vi "FL_Decode_RAW_to_DEC_for_saving.vi"(0 "Sensor board size":string="Small", 1 "IO ports config":bool[](array[boolean])=[TRUE, TRUE, FALSE, FALSE], 2 "Input timestamp":timestamp, 3 "Input string":string, 4 "IO inversion config.":u16, 5 "Error In":errorcluster) -> (6 "Output string leftover":string, 7 "DEC output cluster":T1, 8 "Error Out":errorcluster)   [LabVIEW 2018, in "Tracker.lvlib"]
uses:
  Tracker.lvlib
panel:
  out "TTL ins":bool[](array[boolean])
  out "TTL outs":bool[](array[boolean])
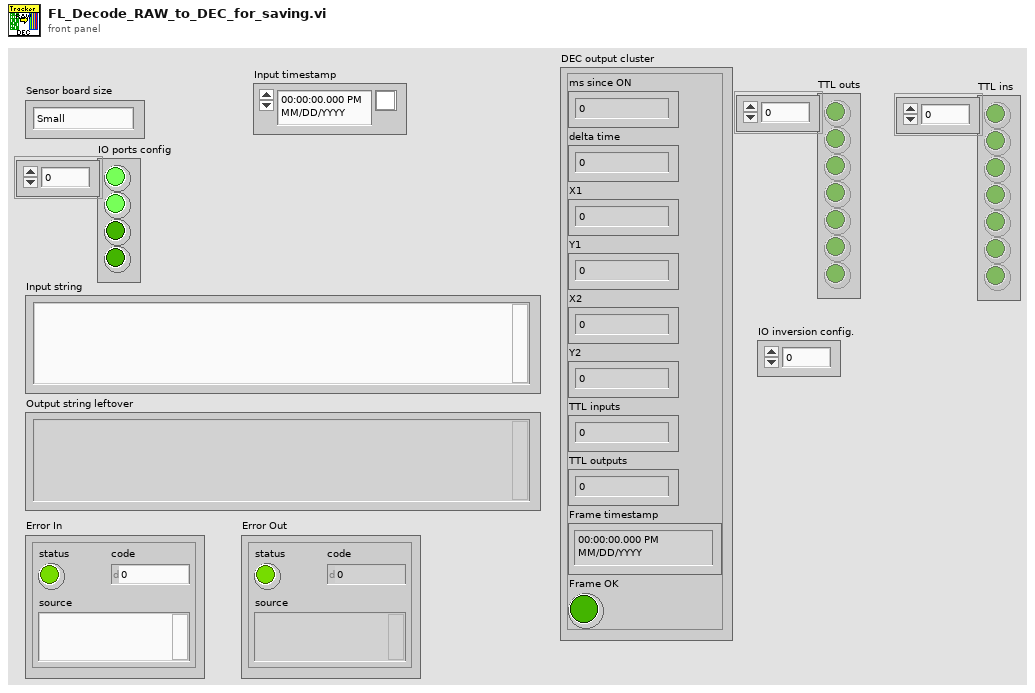
[diagram p1: front panel]
types:
  T1 = cluster{"ms since ON":u32, "delta time":u32, "X1":sgl, "Y1":sgl, "X2":sgl, "Y2":sgl, "TTL inputs":u8, "TTL outputs":u8, "Frame timestamp":timestamp, "Frame OK":bool}
  T2 = cluster{"ms since ON":u32, "delta time":u32, "X1":sgl, "Y1":sgl, "X2":sgl, "Y2":sgl, "TTL IO status":u8, "Frame timestamp":timestamp, "Frame OK":bool}
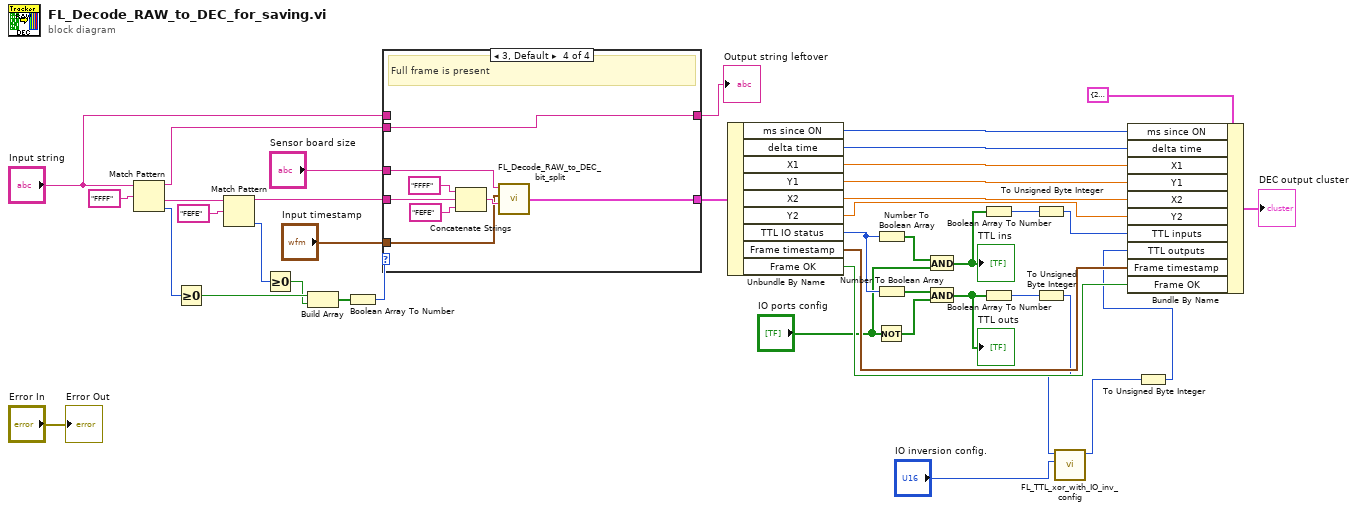
[diagram p0: block diagram]
diagram:
  n1 = Match Pattern(string="Input string", regular expression="FFFF") -> (before substring=w29:string, after substring=w30:string, offset past match=w34:i32)  [unwired: 1 in, 1 out]
  n2 = Greater Or Equal To 0?(x=w34) -> (x >= 0?=w39:bool)
  n3 = Match Pattern(string=w30, regular expression="FEFE") -> (before substring=w33:string, offset past match=w35:i32)  [unwired: 1 in, 2 out]
  n4 = Greater Or Equal To 0?(x=w35) -> (x >= 0?=w38:bool)
  n5 = Build Array(w39, w38) -> (w36:bool[])
  n6 = Boolean Array To Number(Boolean array=w36) -> (number=w37:u32)
  n7 = case shown="3, Default" w37 {
    tunnel: w33 -> [_ _ _ w51]
    tunnel: [_ _ _ w52] -> w25
    tunnel: "Input timestamp" -> [_ _ _ w46]
    tunnel: [w42 w43 w44 w47] -> w31
    tunnel: w29 -> [_ _ _ w47]
    tunnel: "Input string" -> [w42 w43 w44 _]
    tunnel: "Sensor board size" -> [_ _ _ w45]
    frame 0 {
      # "Neither beginning, nor ending of frame is present"
    }
    frame 1 {
      # "Only frame beginning is present"
    }
    frame 2 {
      # "Only frame end is present"
    }
    frame 3, Default {
      # "Full frame is present"
      n8 = Concatenate Strings("FFFF" ("string"), w51, "FEFE" ("string")) -> (w50:string)
      n9 = call "FL_Decode_RAW_to_DEC_bit_split.vi"("Read buffer text to decode"=w50, "Input timestamp"=w46, "Sensor board size"=w45) -> ("DEC output cluster"=w52:T2)  [unwired: 1 in]
    }
  }
  "Output string leftover" <- w31
  n10 = Unbundle By Name(w25) -> ("ms since ON"=w22:u32, "delta time"=w21:u32, "X1"=w20:sgl, "Y1"=w19:sgl, "X2"=w18:sgl, "Y2"=w17:sgl, "TTL IO status"=w13:u8, "Frame timestamp"=w16:timestamp, "Frame OK"=w15:bool)
  n11 = Not(x="IO ports config") -> (.not. x?=w10:bool[])
  n12 = Number To Boolean Array(number=w13) -> (Boolean array=w12:bool[])
  n13 = Number To Boolean Array(number=w13) -> (Boolean array=w14:bool[])
  n14 = And(x=w12, y="IO ports config") -> (x .and. y?=w7:bool[])
  "TTL ins" <- w7
  n15 = And(x=w14, y=w10) -> (x .and. y?=w9:bool[])
  "TTL outs" <- w9
  n16 = Boolean Array To Number(Boolean array=w7) -> (number=w6:u32)
  n17 = Boolean Array To Number(Boolean array=w9) -> (number=w8:u32)
  n18 = To Unsigned Byte Integer(number=w6) -> (unsigned 8bit integer=w5:u8)
  n19 = To Unsigned Byte Integer(number=w8) -> (unsigned 8bit integer=w3:u8)
  n20 = call "FL_TTL_xor_with_IO_inv_config.vi"("IO inversion config."="IO inversion config.", "TTL port(s) config to fire"=w3) -> ("ON config."=w2:u32)  [unwired: 8 in, 1 out]
  n21 = To Unsigned Byte Integer(number=w2) -> (unsigned 8bit integer=w1:u8)
  n22 = Bundle By Name(cluster=T1 {"ms since ON"=21424124, "delta time"=12, "X1"=-25.617287, "Y1"=-34.72222, "X2"=-30.650688, "Y2"=38.869858, "TTL inputs"=4, "TTL outputs"=0, "Frame timestamp"=timestamp(3611917532.9919057 s since 1904-01-01), "Frame OK"=TRUE} ("DEC output cluster"), "ms since ON"=w22, "delta time"=w21, "X1"=w20, "Y1"=w19, "X2"=w18, "Y2"=w17, "TTL inputs"=w5, "TTL outputs"=w1, "Frame timestamp"=w16, "Frame OK"=w15) -> (→"DEC output cluster":T1)
  "Error Out" <- "Error In"
